vi "Remove Actor Ref.vi"(11 "VI Refnum In":refnum<vi>) -> ()   [LabVIEW 2015]
uses:
  Actor Ref Cache Action.ctl
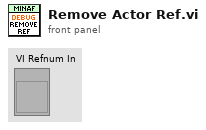
[diagram p1: front panel]
types:
  T1 = typedef "Actor Ref Cache Action.ctl" = enum16{"Clear", "Add Ref", "Remove Ref", "Get All Refs"}
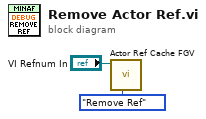
[diagram p0: block diagram]
diagram:
  n1 = call "Actor Ref Cache FGV.vi"("Action"=Actor_Ref_Cache_Action."Remove Ref", "VI Refnum In"="VI Refnum In") -> ()  [unwired: 9 in, 1 out]
